vi "Cholesky decomposition LABVIEW_v1.2.vi"() -> ()   [LabVIEW 2020]
uses:
  <vilib>/Analysis/Matrix/Datatypes/RealMatrix.ctl
  <vilib>/Analysis/baseanly.llb/Real A x B.vi
  <vilib>/Analysis/7linalg.llb/Real Cholesky Factorization.vi
  <vilib>/Analysis/7linalg.llb/Real Transpose Matrix.vi
  <vilib>/Analysis/baseanly.llb/Full Cholesky Factorization.vi
  <vilib>/Analysis/baseanly.llb/Full Real Matrix Cholesky Factorization.vi
  <vilib>/Analysis/Matrix/Numeric/Subtract/Subtract - RM,RM.vi
  <vilib>/Analysis/NI_AALPro.lvlib
  <vilib>/Analysis/Matrix/NI_Matrix.lvlib
  <vilib>/Analysis/NI_AALBase.lvlib
panel:
  out "sum of error":dbl
  out "error":i32
  out "L LABVIEW-FPGA":sgl[][](array[numeric])
  out "L LABVIEW":T1
  out "A input":dbl[][](array[numeric])
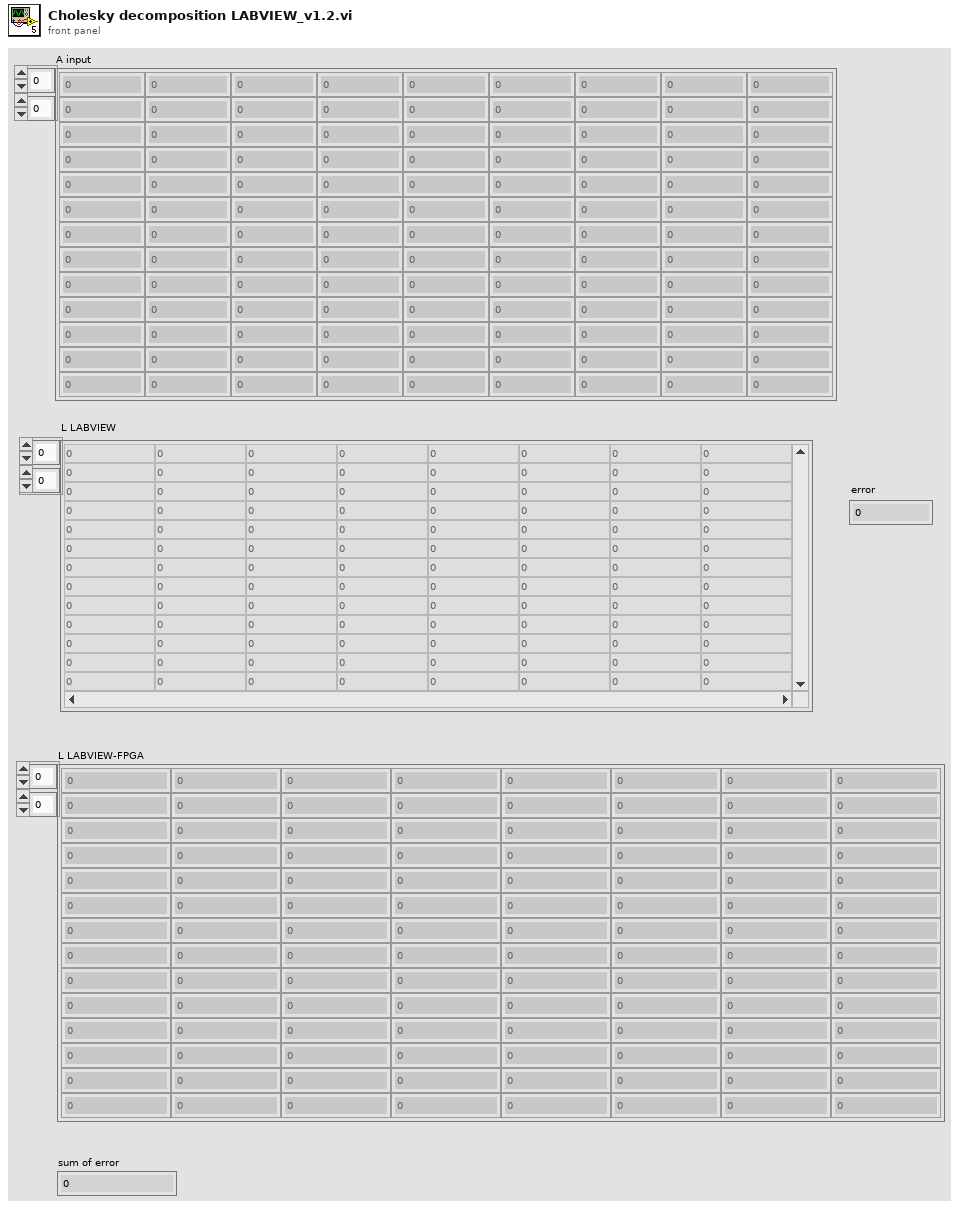
[diagram p1: front panel]
types:
  T1 = typedef "NI_Matrix.lvlib/RealMatrix.ctl" = dbl[][]
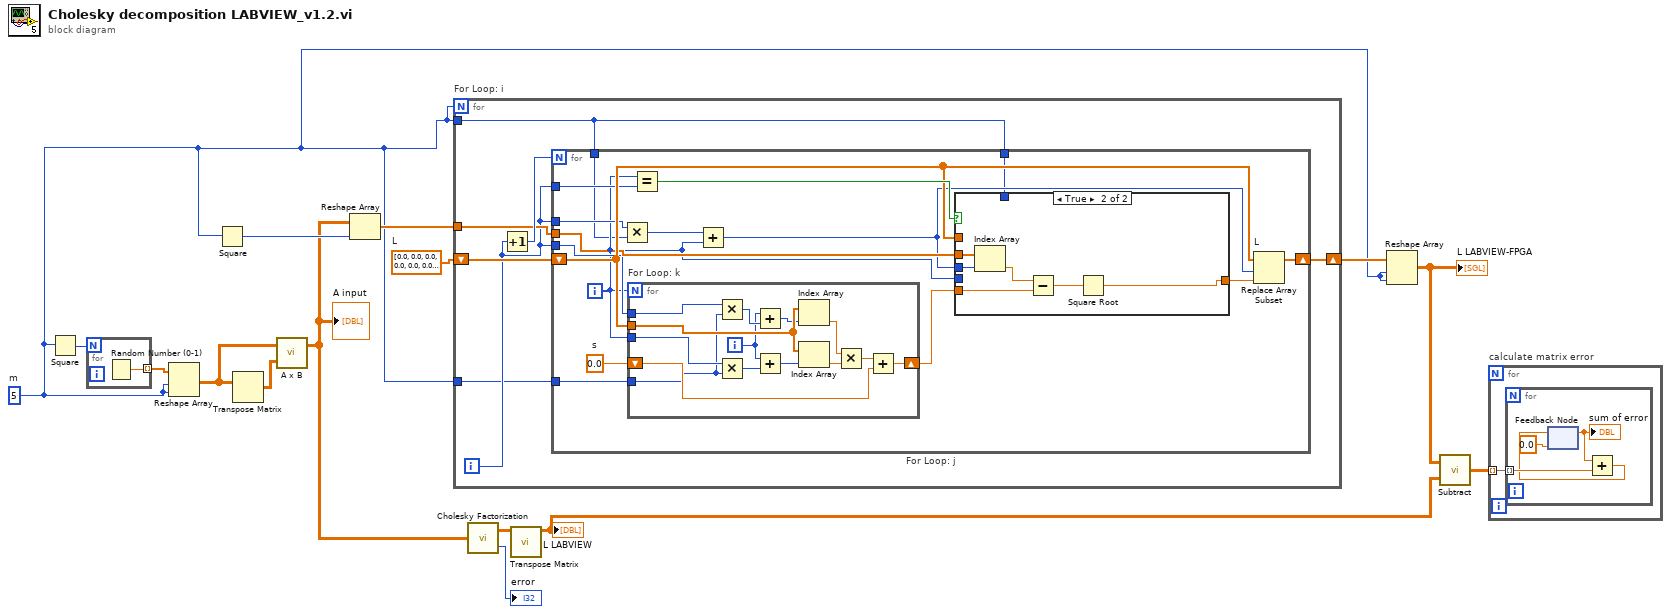
[diagram p0: block diagram]
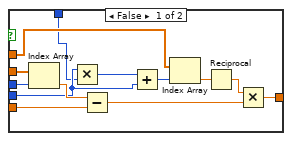
[diagram p2: hidden frame]
diagram:
  w1 = 5  # m
  w15 = sgl[] [0.0, 0.0, 0.0, 0.0, 0.0, 0.0, 0.0, 0.0, 0.0, 0.0, 0.0, 0.0, 0.0, 0.0, 0.0, 0.0, 0.0, 0.0, 0.0, 0.0, 0.0, 0.0, 0.0, 0.0, 0.0, 0.0, 0.0, 0.0, 0.0, 0.0, 0.0, 0.0, 0.0, 0.0, 0.0, 0.0, 0.0, 0.0, 0.0, 0.0, 0.0, 0.0, 0.0, 0.0, 0.0, 0.0, 0.0, 0.0, 0.0, 0.0, 0.0, 0.0, 0.0, 0.0, 0.0, 0.0, 0.0, 0.0, 0.0, 0.0, 0.0, 0.0, 0.0, 0.0, 0.0, 0.0, 0.0, 0.0, 0.0, 0.0, 0.0, 0.0, 0.0, 0.0, 0.0, 0.0, 0.0, 0.0, 0.0, 0.0, 0.0, 0.0, 0.0, 0.0, 0.0, 0.0, 0.0, 0.0, 0.0, 0.0, 0.0, 0.0, 0.0, 0.0, 0.0, 0.0, 0.0, 0.0, 0.0, 0.0, 0.0, 0.0, 0.0, 0.0, 0.0, 0.0, 0.0, 0.0, 0.0, 0.0, 0.0, 0.0, 0.0, 0.0, 0.0, 0.0, 0.0, 0.0, 0.0, 0.0, 0.0, 0.0, 0.0, 0.0, 0.0, 0.0, 0.0, 0.0, 0.0, 0.0, 0.0, 0.0, 0.0, 0.0, 0.0, 0.0, 0.0, 0.0, 0.0, 0.0, 0.0, 0.0, 0.0, 0.0, 0.0, 0.0, 0.0, 0.0, 0.0, 0.0, 0.0, 0.0, 0.0, 0.0, 0.0, 0.0, 0.0, 0.0, 0.0, 0.0, 0.0, 0.0, 0.0, 0.0, 0.0, 0.0, 0.0, 0.0, 0.0, 0.0, 0.0, 0.0, 0.0, 0.0, 0.0, 0.0, 0.0, 0.0, 0.0, 0.0, 0.0, 0.0, 0.0, 0.0, 0.0, 0.0, 0.0, 0.0, 0.0, 0.0, 0.0, 0.0, 0.0, 0.0, 0.0, 0.0, 0.0, 0.0, 0.0, 0.0, 0.0, 0.0, 0.0, 0.0, 0.0, 0.0, 0.0, 0.0, 0.0, 0.0, 0.0, 0.0, 0.0, 0.0, 0.0, 0.0, 0.0, 0.0, 0.0, 0.0, 0.0, 0.0, 0.0, 0.0, 0.0]  # L
  n1 = Square(x=w1) -> (x^2=w6:i32)
  n2 = for {
    N: w6 -> [_]
    tunnel: [w16] -> w5 mode=indexing
    n3 = Random Number (0-1)() -> (number: 0 to 1=w16:dbl)
  }
  n4 = Reshape Array(w5, w1, w1) -> (w3:dbl[][])
  n5 = Square(x=w1) -> (x^2=w11:i32)
  n6 = Transpose Matrix(1:w3) -> (0:w4:dbl[][])
  n7 = call-poly <vilib>:"A x B.vi"("B"=w4, "A"=w3) -> ("A x B"=w2:T1)  [unwired: 1 out]
  "A input" <- w2
  n8 = Reshape Array(w2, w11) -> (w14:dbl[])
  n9 = for "For Loop: i" {
    N: w1 -> [_]
    shift-right: [w21] -> w13
    shift-left: w15 -> [w23]
    tunnel: w14 -> [w20]
    tunnel: w1 -> [w18]
    tunnel: w1 -> [w17]
    i -> [w19]
    n10 = Increment(x=w19) -> (x+1=w22:i32)
    n11 = for "For Loop: j" {
      N: w22 -> [_]
      tunnel: w19 -> [w33]
      shift-right: [w35] -> w21
      shift-left: w23 -> [w34]
      tunnel: w19 -> [w32]
      tunnel: w20 -> [w30]
      tunnel: w19 -> [w28]
      tunnel: w18 -> [w26]
      tunnel: w18 -> [w25]
      tunnel: w17 -> [w24]
      i -> [w27]
      w38 = sgl 0.0  # s
      n12 = Multiply(x=w32, y=w26) -> (x*y=w31:i32)
      n13 = for "For Loop: k" {
        N: w27 -> [_]
        tunnel: w34 -> [w71]
        shift-right: [w67] -> w37
        shift-left: w38 -> [w68]
        tunnel: w28 -> [w66]
        tunnel: w27 -> [w61]
        tunnel: w24 -> [w59]
        i -> [w60]
        n14 = Multiply(x=w66, y=w59) -> (x*y=w65:i32)
        n15 = Multiply(x=w61, y=w59) -> (x*y=w63:i32)
        n16 = Add(x=w60, y=w65) -> (x+y=w64:i32)
        n17 = Add(x=w60, y=w63) -> (x+y=w62:i32)
        n18 = Index Array(array=w71, index=w64) -> (element=w72:sgl)
        n19 = Index Array(array=w71, index=w62) -> (element=w70:sgl)
        n20 = Multiply(x=w72, y=w70) -> (x*y=w69:sgl)
        n21 = Add(x=w69, y=w68) -> (x+y=w67:sgl)
      }
      n22 = Equal?(x=w27, y=w33) -> (x = y?=w39:bool)
      n23 = Add(x=w31, y=w27) -> (x+y=w29:i32)
      n24 = case shown="True" w39 {
        tunnel: w37 -> [w50 w58]
        tunnel: [w49 w56] -> w36
        tunnel: w34 -> [w52 _]
        tunnel: w30 -> [w46 w55]
        tunnel: w29 -> [w45 w54]
        tunnel: w27 -> [w42 _]
        tunnel: w25 -> [w40 _]
        frame False {
          n25 = Index Array(array=w46, index=w45) -> (element=w44:dbl)
          n26 = Multiply(x=w42, y=w40) -> (x*y=w43:i32)
          n27 = Subtract(x=w44, y=w50) -> (x-y=w47:dbl)
          n28 = Add(x=w43, y=w42) -> (x+y=w41:i32)
          n29 = Index Array(array=w52, index=w41) -> (element=w51:sgl)
          n30 = Reciprocal(x=w51) -> (1/x=w48:sgl)
          n31 = Multiply(x=w48, y=w47) -> (x*y=w49:dbl)
        }
        frame True {
          n32 = Index Array(array=w55, index=w54) -> (element=w53:dbl)
          n33 = Subtract(x=w53, y=w58) -> (x-y=w57:dbl)
          n34 = Square Root(x=w57) -> (sqrt(x)=w56:dbl)
        }
      }
      n35 = Replace Array Subset "L"(array=w34, new element=w36, index=w29) -> (w35:sgl[])
    }
  }
  n36 = call-poly <vilib>:"Cholesky Factorization.vi"("A"=w2) -> ("Cholesky"=w10:T1, "error"=→"error":i32)
  n37 = call-poly <vilib>:"Transpose Matrix.vi"("Input Matrix"=w10) -> ("Matrix Transpose"=w7:T1)  [unwired: 9 in, 1 out]
  "L LABVIEW" <- w7
  n38 = Reshape Array(w13, w1, w1) -> (w8:sgl[][])
  "L LABVIEW-FPGA" <- w8
  n39 = call-poly <vilib>:"Subtract.vi"("Real Matrix B"=w7, "Real Matrix A"=w8) -> ("A - B"=w9:T1)
  n40 = for "calculate matrix error" {
    tunnel: w9 -> [w73] mode=indexing
    n41 = for {
      tunnel: w73 -> [w77] mode=indexing
      n42 = feedback #1(0.0) -> (w75:dbl)
      "sum of error" <- w75
      n43 = Add(x=w75, y=w77) -> (x+y=w76:dbl)
      n44 = feedback-in #1(w76) -> ()
    }
  }
